vi "Add.vi"(8 "error in":errorcluster, 11 "UI Data":T1={"Script_Tree"=refnum, "Scripts"=[], "ScriptDetails"={"Script Name"="", "Steps"=[]}, "Current Step"={"StepName"="", "StepDetails"="", "Type"=enum."RELAY_CHANNEL_WRITE"}, "ScriptName"="", "StepName"="", "Children Symbols"=[], "Parrent Symbol"=[], "Configurations:"="", "Config"="", "Scriptno."=0, "PS_Write"={"Set_parameter"=0, "VOLTAGE"="", "CURRENT"="", "OUTPUT"=FALSE, "Delay"=FALSE, "Delay time"=0.0}, "DMM_CONFIG"={"CONFIG PARAMETER"=0, "AUTO RANGE"=FALSE, "RANGE"="", "Delay"=FALSE, "Delay time"=0.0}, "READ_DATAS"={"EQUIPMENT"=0, "PARAMETER"=0, "LSL"=0.0, "USL"=0.0, "RESULT"="", "UNIT"="", "Delay"=FALSE, "Delay time"=0.0}, "Set_Channel_Relay"={"Relay_CH_Array"=[]}, "DAQ_Config"={"AUTO RANGE"=FALSE, "CHANNEL LIST"="", "SELECT Card"=0, "SELECT SLOT"=0, "Function"=0}, "CAN_MSGs_Write"={"Scaling Factor"=1, "Physical value"=0.0, "CAN_Frames"={"CAN_ID"=0, "MSGTYPE"=128, "Payload"=[], "Length"=0}, "Offset value"=0.0, "Framing datas"=[], "CAN_Frame Enable"=FALSE, "Add Signal"=FALSE, "Delete Signal"=FALSE, "Signal Values"=[], "Time(ms)"=0.0, "Repetition"=FALSE, "Delay"=FALSE, "Delay time"=0.0}, "CAN_Read"={"Database"="", "Signal"="", "BYTES"=[], "ReadPayload"=[], "String_Data"="", "ReadValue"=0.0, "CANID"=0, "SERVICE ID"=0, "SUB-SERVICE ID"=0, "DELAY "=FALSE, "Delay time(ms)"=0.0}, "Camera"={"Trigger"=FALSE, "Prog No."="", "Delay"=FALSE, "Delay time"=0.0, "Storage"="", "Col no."="", "Row no."=""}, "Tab Control"=refnum, "MCU Flashing"={"Result Path"=path "", "Result"=""}, "Noeway_Flashing"={"Neoway_Firmware"=path "", "RESULT STRING"="", "Delay"=FALSE, "Delay time"=0.0}, "SSL"={"SSL_EXE"=path "", "RESULT STRING"="", "Delay"=FALSE, "Delay time"=0.0}} {"CAN_Read"."SUB-SERVICE ID" format="%.0x"; "CAN_Read"."SERVICE ID" format="%.0x"; "CAN_Read"."CANID" format="%.0x"; "CAN_Read"."ReadPayload" format="%.0x"; "CAN_MSGs_Write"."CAN_Frames"."Payload" format="%.0x"; "CAN_MSGs_Write"."CAN_Frames"."MSGTYPE" items=["STATUS"=128, "EXTENDED"=2, "RTR"=1, "DATA MSG"=0]; "CAN_MSGs_Write"."CAN_Frames"."CAN_ID" format="%.0x"; "DAQ_Config"."Function" items=["Voltage DC", "Voltage AC", "Current DC", "Current AC", "Resistance", "4-wire Resistance", "Diode", "Capacitance", "Temperature", "Continuity", "Frequency", "Period", "Voltage Ratio", "Digitize Voltage", "Digitize Current"]; "DAQ_Config"."SELECT SLOT" items=["Slot 1", "Slot 2"]; "DAQ_Config"."SELECT Card" items=["7708", "7700"]; "Set_Channel_Relay"."Relay_CH_Array"."OUTPUT_Relay_Channels" items=["CONN_SUPPLY_%d_FCT", "HB_CONN_%d_FCT", "L_IND_CONN_%d_FCT", "R_IND_CONN_%d_FCT", "SW1_%d_FCT", "SW2_%d_FCT", "CAN_H_%d_FCT", "CAN_L_%d_FCT", "CYLINDER_ON/OFF_%d_FCT", "SPARE_1_%d_FCT", "SPARE_2_%d_FCT", "Tower Red", "Tower Amber", "Tower Green", "Tower Buzzer", "SLIMRELAY_DUT_%d_FCT", "GND_DMM_%d_EOL", "CAN_H_RES_%d_EOL", "CAN_L_RES_%d_EOL", "L_IND_RES_%d_EOL", "R_IND_RES_%d_EOL", "HB_CONN_DMM_%d_EOL", "14V_RES_%d_EOL", "CAN_L_(DMM-)_%d_EOL", "CAN_H_%d_EOL", "CAN_L_%d_EOL", "14V_%d_EOL", "GND_%d_EOL", "HB_CONN_%d_EOL", "L_IND_%d_EOL", "R_IND_%d_EOL", "CYLINDER_DUT_%d_EOL", "CYL_PB_1_%d_EOL", "CYL_PB_2_%d_EOL", "DUT_PASS_%d_EOL", "DUT_FAIL_%d_EOL", "SPARE1_%d_EOL", "Tower Red_EOL", "Tower Amber_EOL", "Tower Green_EOL", "Tower Buzzer_EOL"]; "READ_DATAS"."PARAMETER" items=["SET_VOLTAGE", "SET_CURRENT", "OUTPUT VOLTAGE", "OUTPUT CURRENT", "RESISTANCE", "OUTPUT POWER", "CAMERA", "SSL_Check"]; "READ_DATAS"."EQUIPMENT" items=["POWER SUPPLY", "DMM", "DAQ", "CAMERA"]; "DMM_CONFIG"."CONFIG PARAMETER" items=["VOLTAGE", "CURRENT", "RESISTANCE", "POWER"]; "PS_Write"."Set_parameter" items=["Set_Voltage", "Set_current", "Output"]}) -> (0 "error out":errorcluster, 1 "Draw":bool, 2 "Valid":bool, 3 "UI Data out":T1={"Script_Tree"=refnum, "Scripts"=[], "ScriptDetails"={"Script Name"="", "Steps"=[]}, "Current Step"={"StepName"="", "StepDetails"="", "Type"=enum."RELAY_CHANNEL_WRITE"}, "ScriptName"="", "StepName"="", "Children Symbols"=[], "Parrent Symbol"=[], "Configurations:"="", "Config"="", "Scriptno."=0, "PS_Write"={"Set_parameter"=0, "VOLTAGE"="", "CURRENT"="", "OUTPUT"=FALSE, "Delay"=FALSE, "Delay time"=0.0}, "DMM_CONFIG"={"CONFIG PARAMETER"=0, "AUTO RANGE"=FALSE, "RANGE"="", "Delay"=FALSE, "Delay time"=0.0}, "READ_DATAS"={"EQUIPMENT"=0, "PARAMETER"=0, "LSL"=0.0, "USL"=0.0, "RESULT"="", "UNIT"="", "Delay"=FALSE, "Delay time"=0.0}, "Set_Channel_Relay"={"Relay_CH_Array"=[]}, "DAQ_Config"={"AUTO RANGE"=FALSE, "CHANNEL LIST"="", "SELECT Card"=0, "SELECT SLOT"=0, "Function"=0}, "CAN_MSGs_Write"={"Scaling Factor"=1, "Physical value"=0.0, "CAN_Frames"={"CAN_ID"=0, "MSGTYPE"=128, "Payload"=[], "Length"=0}, "Offset value"=0.0, "Framing datas"=[], "CAN_Frame Enable"=FALSE, "Add Signal"=FALSE, "Delete Signal"=FALSE, "Signal Values"=[], "Time(ms)"=0.0, "Repetition"=FALSE, "Delay"=FALSE, "Delay time"=0.0}, "CAN_Read"={"Database"="", "Signal"="", "BYTES"=[], "ReadPayload"=[], "String_Data"="", "ReadValue"=0.0, "CANID"=0, "SERVICE ID"=0, "SUB-SERVICE ID"=0, "DELAY "=FALSE, "Delay time(ms)"=0.0}, "Camera"={"Trigger"=FALSE, "Prog No."="", "Delay"=FALSE, "Delay time"=0.0, "Storage"="", "Col no."="", "Row no."=""}, "Tab Control"=refnum, "MCU Flashing"={"Result Path"=path "", "Result"=""}, "Noeway_Flashing"={"Neoway_Firmware"=path "", "RESULT STRING"="", "Delay"=FALSE, "Delay time"=0.0}, "SSL"={"SSL_EXE"=path "", "RESULT STRING"="", "Delay"=FALSE, "Delay time"=0.0}} {"CAN_Read"."SUB-SERVICE ID" format="%.0x"; "CAN_Read"."SERVICE ID" format="%.0x"; "CAN_Read"."CANID" format="%.0x"; "CAN_Read"."ReadPayload" format="%.0x"; "CAN_MSGs_Write"."CAN_Frames"."Payload" format="%.0x"; "CAN_MSGs_Write"."CAN_Frames"."MSGTYPE" items=["STATUS"=128, "EXTENDED"=2, "RTR"=1, "DATA MSG"=0]; "CAN_MSGs_Write"."CAN_Frames"."CAN_ID" format="%.0x"; "DAQ_Config"."Function" items=["Voltage DC", "Voltage AC", "Current DC", "Current AC", "Resistance", "4-wire Resistance", "Diode", "Capacitance", "Temperature", "Continuity", "Frequency", "Period", "Voltage Ratio", "Digitize Voltage", "Digitize Current"]; "DAQ_Config"."SELECT SLOT" items=["Slot 1", "Slot 2"]; "DAQ_Config"."SELECT Card" items=["7708", "7700"]; "Set_Channel_Relay"."Relay_CH_Array"."OUTPUT_Relay_Channels" items=["CONN_SUPPLY_%d_FCT", "HB_CONN_%d_FCT", "L_IND_CONN_%d_FCT", "R_IND_CONN_%d_FCT", "SW1_%d_FCT", "SW2_%d_FCT", "CAN_H_%d_FCT", "CAN_L_%d_FCT", "CYLINDER_ON/OFF_%d_FCT", "SPARE_1_%d_FCT", "SPARE_2_%d_FCT", "Tower Red", "Tower Amber", "Tower Green", "Tower Buzzer", "SLIMRELAY_DUT_%d_FCT", "GND_DMM_%d_EOL", "CAN_H_RES_%d_EOL", "CAN_L_RES_%d_EOL", "L_IND_RES_%d_EOL", "R_IND_RES_%d_EOL", "HB_CONN_DMM_%d_EOL", "14V_RES_%d_EOL", "CAN_L_(DMM-)_%d_EOL", "CAN_H_%d_EOL", "CAN_L_%d_EOL", "14V_%d_EOL", "GND_%d_EOL", "HB_CONN_%d_EOL", "L_IND_%d_EOL", "R_IND_%d_EOL", "CYLINDER_DUT_%d_EOL", "CYL_PB_1_%d_EOL", "CYL_PB_2_%d_EOL", "DUT_PASS_%d_EOL", "DUT_FAIL_%d_EOL", "SPARE1_%d_EOL", "Tower Red_EOL", "Tower Amber_EOL", "Tower Green_EOL", "Tower Buzzer_EOL"]; "READ_DATAS"."PARAMETER" items=["SET_VOLTAGE", "SET_CURRENT", "OUTPUT VOLTAGE", "OUTPUT CURRENT", "RESISTANCE", "OUTPUT POWER", "CAMERA", "SSL_Check"]; "READ_DATAS"."EQUIPMENT" items=["POWER SUPPLY", "DMM", "DAQ", "CAMERA"]; "DMM_CONFIG"."CONFIG PARAMETER" items=["VOLTAGE", "CURRENT", "RESISTANCE", "POWER"]; "PS_Write"."Set_parameter" items=["Set_Voltage", "Set_current", "Output"]})   [LabVIEW 2024, in "Setting_Screen.lvlib"]
uses:
  Setting_Screen.lvlib
  controls/Setting_Screen UI Data.ctl
  ScriptDetails.ctl
  CurrentStep.ctl
  StepType.ctl
  PS_WRITE.ctl
  PS_set.ctl
  DMM_CONFIG.ctl
  READ_DATAS.ctl
  READ_EQP.ctl
  READ_PARA.ctl
  Relay_Channel_Array.ctl
  Common_plc_DOs.ctl
  DAQ_Config.ctl
  PCANusb_DTU/support/CAN_MSGs.ctl
  PCANusb_DTU/support/CAN_Frames_ctrl.ctl
  PCANusb_DTU/support/Framing datas.ctl
  PCANusb_DTU/support/CAN_Read.ctl
  Camera.ctl
  Steptab.ctl
  MCU_Flashing/support/MCU_ctrl.ctl
  Neoway ctl.ctl
  SSL.ctl
  PCANusb_DTU/PCANusb_DTU.lvlib
  MCU_Flashing/MCU_Flashing.lvlib
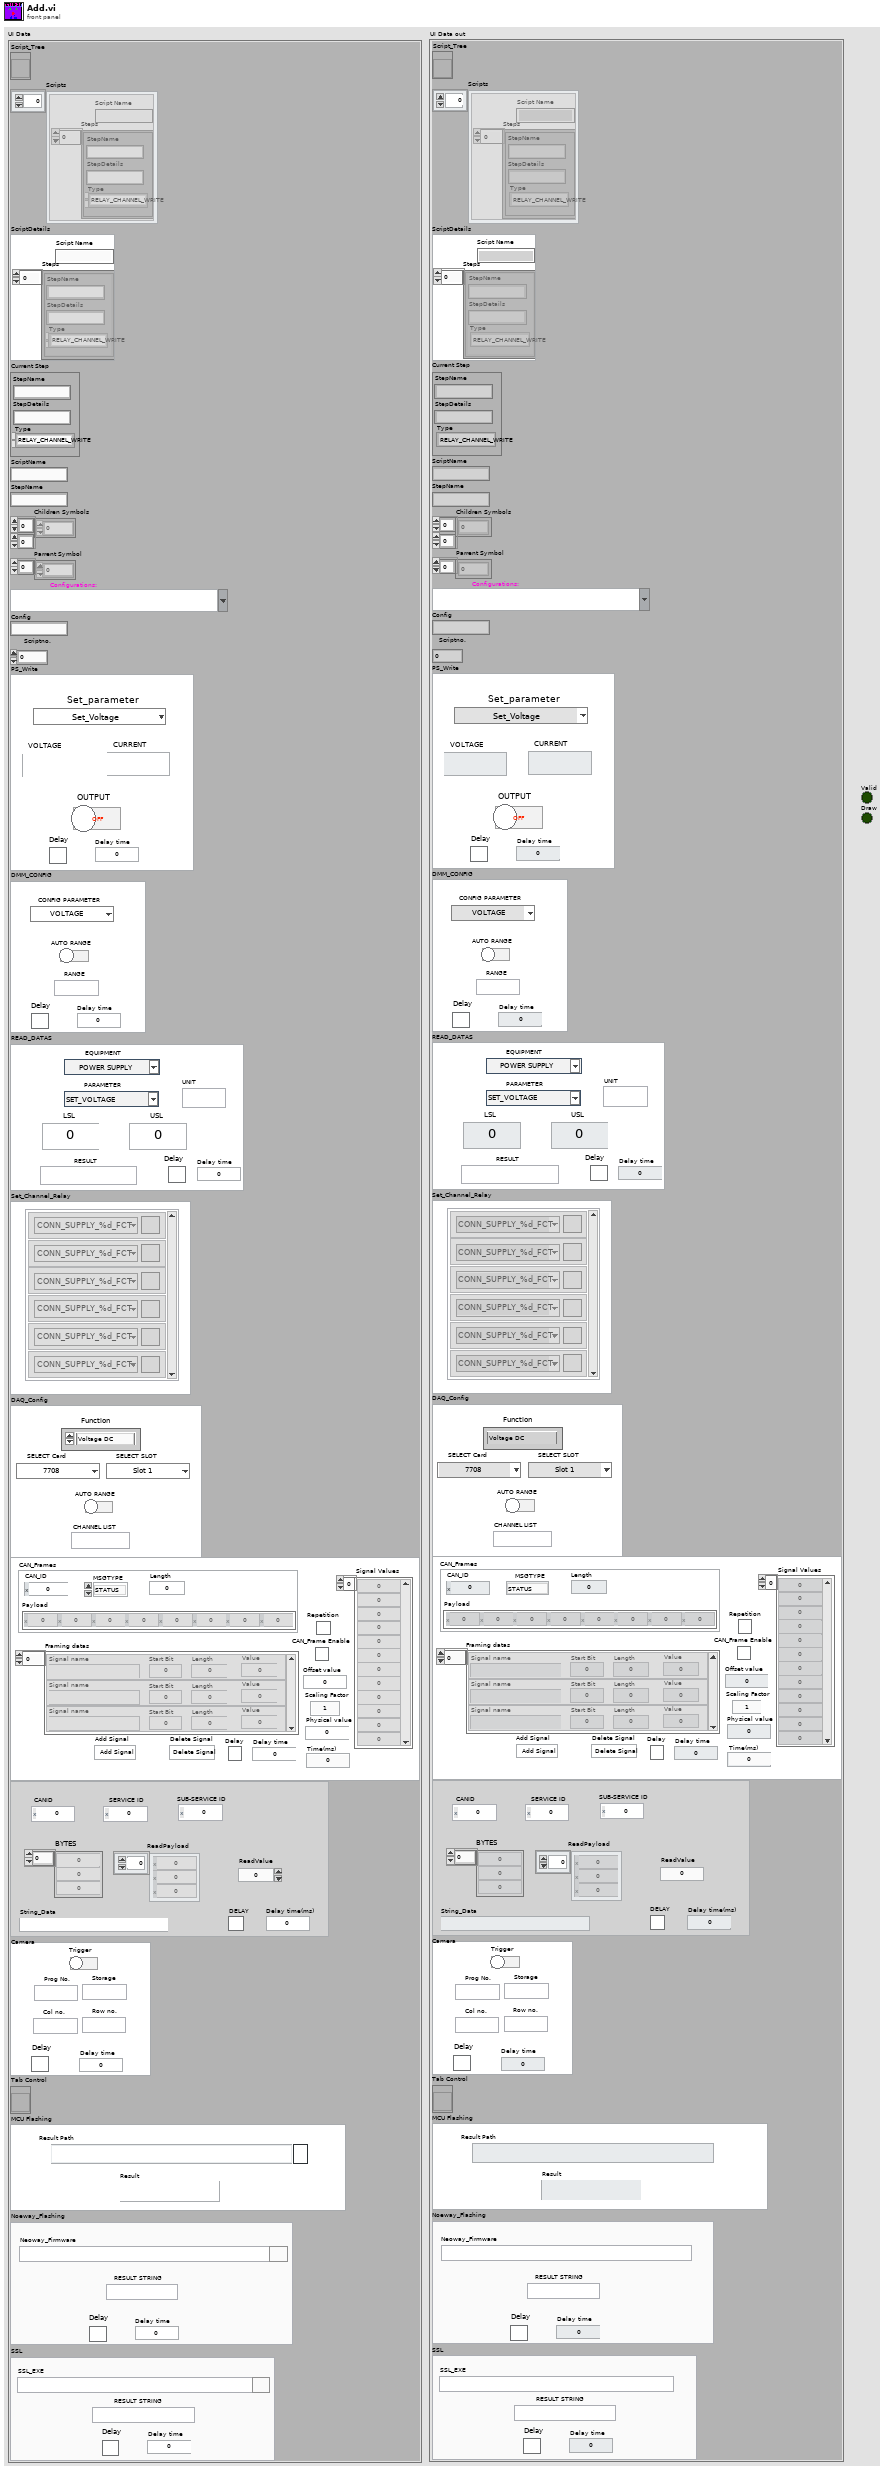
[diagram p1: front panel]
types:
  T1 = typedef "Setting_Screen.lvlib/Setting_Screen UI Data.ctl" = cluster{"Script_Tree":refnum<vi>, "Scripts":T2[], "ScriptDetails":T2, "Current Step":T3, "ScriptName":string, "StepName":string, "Children Symbols":i32[][], "Parrent Symbol":i32[], "Configurations:":string, "Config":string, "Scriptno.":i32, "PS_Write":T5, "DMM_CONFIG":T7, "READ_DATAS":T8, "Set_Channel_Relay":T11, "DAQ_Config":T13, "CAN_MSGs_Write":T14, "CAN_Read":T17, "Camera":T18, "Tab Control":refnum<vi>, "MCU Flashing":T19, "Noeway_Flashing":T20, "SSL":T21}
  T2 = typedef "Setting_Screen.lvlib/ScriptDetails.ctl" = cluster{"Script Name":string, "Steps":T3[]}
  T3 = typedef "Setting_Screen.lvlib/CurrentStep.ctl" = cluster{"StepName":string, "StepDetails":string, "Type":T4}
  T4 = typedef "Setting_Screen.lvlib/StepType.ctl" = enum16{"RELAY_CHANNEL_WRITE", "PS_WRITE", "READ_DATA", "DMM_CONFIG", "DAQ_CONFIG", "PCAN_Read", "PCAN_Write", "Camera", "MCU_Flashing", "Noeway_Flashing", "SSL_Certification"}
  T5 = typedef "Setting_Screen.lvlib/PS_WRITE.ctl" = cluster{"Set_parameter":T6, "VOLTAGE":string, "CURRENT":string, "OUTPUT":bool, "Delay":bool, "Delay time":dbl}
  T6 = typedef "Setting_Screen.lvlib/PS_set.ctl" = u16
  T7 = typedef "Setting_Screen.lvlib/DMM_CONFIG.ctl" = cluster{"CONFIG PARAMETER":u16, "AUTO RANGE":bool, "RANGE":string, "Delay":bool, "Delay time":dbl}
  T8 = typedef "Setting_Screen.lvlib/READ_DATAS.ctl" = cluster{"EQUIPMENT":T9, "PARAMETER":T10, "LSL":dbl, "USL":dbl, "RESULT":string, "UNIT":string, "Delay":bool, "Delay time":dbl}
  T9 = typedef "Setting_Screen.lvlib/READ_EQP.ctl" = u16
  T10 = typedef "Setting_Screen.lvlib/READ_PARA.ctl" = u16
  T11 = typedef "Setting_Screen.lvlib/Relay_Channel_Array.ctl" = cluster{"Relay_CH_Array":cluster{"OUTPUT_Relay_Channels":T12, "On/Off":bool}[]}
  T12 = typedef "Setting_Screen.lvlib/Common_plc_DOs.ctl" = u16
  T13 = typedef "Setting_Screen.lvlib/DAQ_Config.ctl" = cluster{"AUTO RANGE":bool, "CHANNEL LIST":string, "SELECT Card":u16, "SELECT SLOT":u16, "Function":i32}
  T14 = typedef "PCANusb_DTU.lvlib/CAN_MSGs.ctl" = cluster{"Scaling Factor":u16, "Physical value":dbl, "CAN_Frames":T15, "Offset value":dbl, "Framing datas":T16[], "CAN_Frame Enable":bool, "Add Signal":bool, "Delete Signal":bool, "Signal Values":dbl[], "Time(ms)":dbl, "Repetition":bool, "Delay":bool, "Delay time":dbl}
  T15 = typedef "PCANusb_DTU.lvlib/CAN_Frames_ctrl.ctl" = cluster{"CAN_ID":u32, "MSGTYPE":u8, "Payload":u8[], "Length":u8}
  T16 = typedef "PCANusb_DTU.lvlib/Framing datas.ctl" = cluster{"Signal name":string, "Start Bit":u8, "Length":u8, "Value":u16}
  T17 = typedef "PCANusb_DTU.lvlib/CAN_Read.ctl" = cluster{"Database":refnum<k21>, "Signal":refnum<k21>, "BYTES":u32[], "ReadPayload":u8[], "String_Data":string, "ReadValue":dbl, "CANID":u32, "SERVICE ID":u32, "SUB-SERVICE ID":u32, "DELAY ":bool, "Delay time(ms)":dbl}
  T18 = typedef "Setting_Screen.lvlib/Camera.ctl" = cluster{"Trigger":bool, "Prog No.":string, "Delay":bool, "Delay time":dbl, "Storage":string, "Col no.":string, "Row no.":string}
  T19 = typedef "MCU_Flashing.lvlib/MCU_ctrl.ctl" = cluster{"Result Path":path, "Result":string}
  T20 = typedef "Neoway ctl.ctl" = cluster{"Neoway_Firmware":path, "RESULT STRING":string, "Delay":bool, "Delay time":dbl}
  T21 = typedef "SSL.ctl" = cluster{"SSL_EXE":path, "RESULT STRING":string, "Delay":bool, "Delay time":dbl}
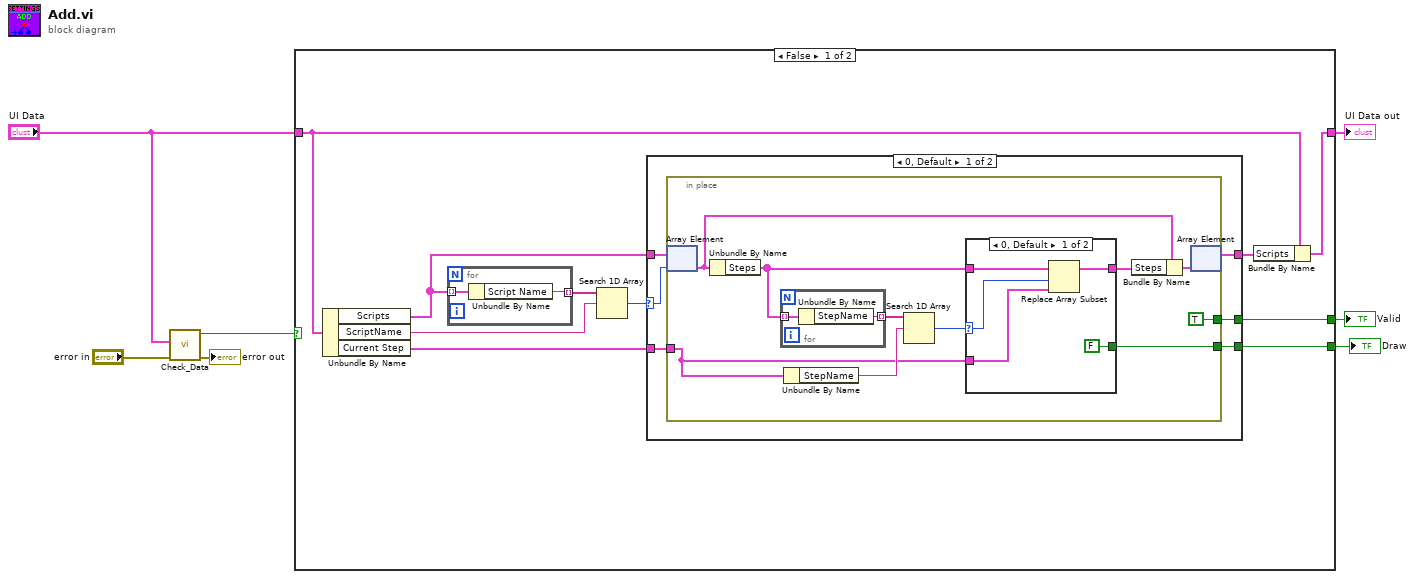
[diagram p0: block diagram]
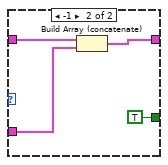
[diagram p2: hidden frame]
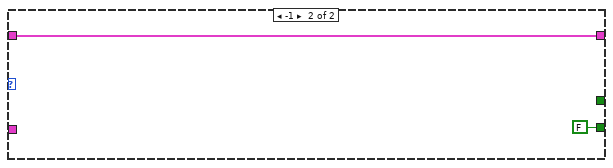
[diagram p3: hidden frame]
diagram:
  n1 = call "Check_Data.vi"("error constant"="error in", "UI Data"="UI Data") -> ("error constant 2"=→"error out":errorcluster, "Fail?"=w6:bool)  [unwired: 8 in]
  n2 = case shown="False" w6 {
    tunnel: "UI Data" -> [w17 w49]
    tunnel: [w12 w49] -> w3
    tunnel: [w9 _] -> w2
    tunnel: [w8 _] -> w1
    frame False {
      n3 = Unbundle By Name(w17) -> ("Scripts"=w13:T2[], "ScriptName"=w14:string, "Current Step"=w10:T3)
      n4 = for {
        tunnel: w13 -> [w48] mode=indexing
        tunnel: [w47] -> w15 mode=indexing
        n5 = Unbundle By Name(w48) -> ("Script Name"=w47:string)
      }
      n6 = Search 1D Array(1D array=w15, element=w14) -> (index of element=w16:i32)  [unwired: 1 in]
      n7 = case shown="0, Default" w16 {
        selector: w16 -> [w23 _]
        tunnel: w13 -> [w22 w46]
        tunnel: [w21 w46] -> w11
        tunnel: w10 -> [w20 _]
        tunnel: [w19 _] -> w9
        tunnel: [w18 FALSE] -> w8
        frame 0, Default {
          n8 = in-place {
            in-place-border: w20 -> [w29]
            in-place-border: [TRUE] -> w19
            in-place-border: [w24] -> w18
            n9 = in-place-array #1(w22, w23) -> (w28:T2)
            n10 = Unbundle By Name(w28) -> ("Steps"=w30:T3[])
            n11 = for {
              tunnel: w30 -> [w44] mode=indexing
              tunnel: [w43] -> w33 mode=indexing
              n12 = Unbundle By Name(w44) -> ("StepName"=w43:string)
            }
            n13 = Unbundle By Name(w29) -> ("StepName"=w32:string)
            n14 = Search 1D Array(1D array=w33, element=w32) -> (index of element=w31:i32)  [unwired: 1 in]
            n15 = case shown="0, Default" w31 {
              selector: w31 -> [w37 _]
              tunnel: w30 -> [w38 w42]
              tunnel: [w36 w41] -> w27
              tunnel: w29 -> [w35 w40]
              tunnel: [FALSE TRUE] -> w24
              frame 0, Default {
                n16 = Replace Array Subset(array=w38, new element=w35, index=w37) -> (w36:T3[])
              }
              frame -1 {
                n17 = Build Array (concatenate)(w42, w40) -> (w41:T3[])
              }
            }
            n18 = Bundle By Name(cluster=w28, "Steps"=w27) -> (w26:T2)
            n19 = in-place-array #1(w26) -> (w21:T2[])  [unwired: 1 out]
          }
        }
        frame -1 {
        }
      }
      n20 = Bundle By Name(cluster=w17, "Scripts"=w11) -> (w12:T1)
    }
    frame True {
    }
  }
  "UI Data out" <- w3
  "Valid" <- w2
  "Draw" <- w1
